vi "NEO Set Pod Setpoints.vi"(6 "Operation":T2, 8 "Steer Angles (degrees)":T3, 9 "Drive Velocities (ft/s)":T3, 10 "Pod Setpoints (ft/s and deg)":T16, 11 "Swerve Drive":T5={"Drive Motors (NEO)"={"Left Front"={"DeviceStatus"={"status"=FALSE, "code"=0, "source"=""}, "Type"=enum."PWM", "PWM"={"PWM Channel"=enum."Invalid", "DeadBand"={"Name"="", "maxPositivePwm"=0, "minPositivePwm"=0, "centerPwm"=0, "maxNegativePwm"=0, "minNegativePwm"=0, "angularRange"=0}}, "CAN"={"Device Number"=0, "SetOutput VI Ref"=variant, "GetOutput VI Ref"=variant, "Enable VI Ref"=variant, "Disable VI Ref"=variant, "Data"=variant}, "Invert"=FALSE, "DIO PWM"={"PWM \"Enable\" Channel"=enum."Invalid", "DIOChannel"=enum."Invalid", "PWM Rate"=0.0}}, "Left Back"={"DeviceStatus"={"status"=FALSE, "code"=0, "source"=""}, "Type"=enum."PWM", "PWM"={"PWM Channel"=enum."Invalid", "DeadBand"={"Name"="", "maxPositivePwm"=0, "minPositivePwm"=0, "centerPwm"=0, "maxNegativePwm"=0, "minNegativePwm"=0, "angularRange"=0}}, "CAN"={"Device Number"=0, "SetOutput VI Ref"=variant, "GetOutput VI Ref"=variant, "Enable VI Ref"=variant, "Disable VI Ref"=variant, "Data"=variant}, "Invert"=FALSE, "DIO PWM"={"PWM \"Enable\" Channel"=enum."Invalid", "DIOChannel"=enum."Invalid", "PWM Rate"=0.0}}, "Right Front"={"DeviceStatus"={"status"=FALSE, "code"=0, "source"=""}, "Type"=enum."PWM", "PWM"={"PWM Channel"=enum."Invalid", "DeadBand"={"Name"="", "maxPositivePwm"=0, "minPositivePwm"=0, "centerPwm"=0, "maxNegativePwm"=0, "minNegativePwm"=0, "angularRange"=0}}, "CAN"={"Device Number"=0, "SetOutput VI Ref"=variant, "GetOutput VI Ref"=variant, "Enable VI Ref"=variant, "Disable VI Ref"=variant, "Data"=variant}, "Invert"=FALSE, "DIO PWM"={"PWM \"Enable\" Channel"=enum."Invalid", "DIOChannel"=enum."Invalid", "PWM Rate"=0.0}}, "Right Back"={"DeviceStatus"={"status"=FALSE, "code"=0, "source"=""}, "Type"=enum."PWM", "PWM"={"PWM Channel"=enum."Invalid", "DeadBand"={"Name"="", "maxPositivePwm"=0, "minPositivePwm"=0, "centerPwm"=0, "maxNegativePwm"=0, "minNegativePwm"=0, "angularRange"=0}}, "CAN"={"Device Number"=0, "SetOutput VI Ref"=variant, "GetOutput VI Ref"=variant, "Enable VI Ref"=variant, "Disable VI Ref"=variant, "Data"=variant}, "Invert"=FALSE, "DIO PWM"={"PWM \"Enable\" Channel"=enum."Invalid", "DIOChannel"=enum."Invalid", "PWM Rate"=0.0}}}, "Steer Motors (NEO)"={"Left Front"={"DeviceStatus"={"status"=FALSE, "code"=0, "source"=""}, "Type"=enum."PWM", "PWM"={"PWM Channel"=enum."Invalid", "DeadBand"={"Name"="", "maxPositivePwm"=0, "minPositivePwm"=0, "centerPwm"=0, "maxNegativePwm"=0, "minNegativePwm"=0, "angularRange"=0}}, "CAN"={"Device Number"=0, "SetOutput VI Ref"=variant, "GetOutput VI Ref"=variant, "Enable VI Ref"=variant, "Disable VI Ref"=variant, "Data"=variant}, "Invert"=FALSE, "DIO PWM"={"PWM \"Enable\" Channel"=enum."Invalid", "DIOChannel"=enum."Invalid", "PWM Rate"=0.0}}, "Left Back"={"DeviceStatus"={"status"=FALSE, "code"=0, "source"=""}, "Type"=enum."PWM", "PWM"={"PWM Channel"=enum."Invalid", "DeadBand"={"Name"="", "maxPositivePwm"=0, "minPositivePwm"=0, "centerPwm"=0, "maxNegativePwm"=0, "minNegativePwm"=0, "angularRange"=0}}, "CAN"={"Device Number"=0, "SetOutput VI Ref"=variant, "GetOutput VI Ref"=variant, "Enable VI Ref"=variant, "Disable VI Ref"=variant, "Data"=variant}, "Invert"=FALSE, "DIO PWM"={"PWM \"Enable\" Channel"=enum."Invalid", "DIOChannel"=enum."Invalid", "PWM Rate"=0.0}}, "Right Front"={"DeviceStatus"={"status"=FALSE, "code"=0, "source"=""}, "Type"=enum."PWM", "PWM"={"PWM Channel"=enum."Invalid", "DeadBand"={"Name"="", "maxPositivePwm"=0, "minPositivePwm"=0, "centerPwm"=0, "maxNegativePwm"=0, "minNegativePwm"=0, "angularRange"=0}}, "CAN"={"Device Number"=0, "SetOutput VI Ref"=variant, "GetOutput VI Ref"=variant, "Enable VI Ref"=variant, "Disable VI Ref"=variant, "Data"=variant}, "Invert"=FALSE, "DIO PWM"={"PWM \"Enable\" Channel"=enum."Invalid", "DIOChannel"=enum."Invalid", "PWM Rate"=0.0}}, "Right Back"={"DeviceStatus"={"status"=FALSE, "code"=0, "source"=""}, "Type"=enum."PWM", "PWM"={"PWM Channel"=enum."Invalid", "DeadBand"={"Name"="", "maxPositivePwm"=0, "minPositivePwm"=0, "centerPwm"=0, "maxNegativePwm"=0, "minNegativePwm"=0, "angularRange"=0}}, "CAN"={"Device Number"=0, "SetOutput VI Ref"=variant, "GetOutput VI Ref"=variant, "Enable VI Ref"=variant, "Disable VI Ref"=variant, "Data"=variant}, "Invert"=FALSE, "DIO PWM"={"PWM \"Enable\" Channel"=enum."Invalid", "DIOChannel"=enum."Invalid", "PWM Rate"=0.0}}}, "Pigeon2"={"DeviceStatus"={"status"=FALSE, "code"=0, "source"=""}, "Device Number"=0, "Type"=352321536, "Device ID"=0, "Handle"=0, "UsageFrame"=0, "Library Path"=path ""}, "Radii (ft)"={"Left Front Position"=[], "Left Back Position"=[], "Right Front Position"=[], "Right Back Position"=[]}} {"Radii (ft)"."Right Back Position" format="%.2f"; "Radii (ft)"."Right Front Position" format="%.2f"; "Radii (ft)"."Left Back Position" format="%.2f"; "Radii (ft)"."Left Front Position" format="%.2f"; "Pigeon2"."Type" items=["CAN"=352321536, "TalonSRX"=33554432]}) -> ()   [LabVIEW 2023]
uses:
  Type Definitions/Data/Pod Setpoints.ctl
  Type Definitions/Hardware/Swerve Drives/(NEO-NEO-ThroughBore-Pigeon2) Swerve.ctl
  Type Definitions/Hardware/4 Motor Sets/(NEO & NEO 550) 4 Motor Set.ctl
  <vilib>/Rock Robotics/WPI/MotorControl/WPI_MotorControlDeviceRef.ctl
  <vilib>/Rock Robotics/WPI/MotorControl/WPI_MotorControlType.ctl
  <vilib>/Rock Robotics/SystemInterfaces/DIO/FPGA_DIOPWMChannel.ctl
  <vilib>/Rock Robotics/WPI/PWM/WPI_PWMDeadband.ctl
  <vilib>/Rock Robotics/SystemInterfaces/DIO/FPGA_DIOChannel.ctl
  <vilib>/Rock Robotics/WPI/ThirdParty/Phoenix-LabVIEW/Pigeon IMU/CTRE_PigeonIMU_DeviceRef.ctl
  <vilib>/Rock Robotics/WPI/ThirdParty/Phoenix-LabVIEW/Pigeon IMU/CTRE_PigeonIMU_ConnectionType.ctl
  Type Definitions/Data/Pod Positions.ctl
  Robot Code/Drive/Implementation/Drive Operations.ctl
  <vilib>/Rock Robotics/WPI/ThirdParty/REV Robotics/REVLib/Typedef/Spark MAX Control Type.ctl
  4b768f86-8279-4062-bf26-12cbbaf62c6c.vi
panel:
  out "Arbitrary":T1
  in  "PID Constants":T4={"P Gain"=0.0, "I Gain"=0.0, "D Gain"=0.0, "F Gain"=0.0, "I Zone"=0.0, "Min Output"=-1.0, "Max Output"=1.0}
  in  "Motor Type":enum16{"Drive", "Steer"}(ring)
  in  "Motor Position":T15(ring)
  out "PID Graph":cluster{"Left Front":dbl, "Theta":dbl}(graph)
  out "Values":cluster{"Actual":dbl, "Setpoint":dbl}
  in  "Debug Mode?":bool
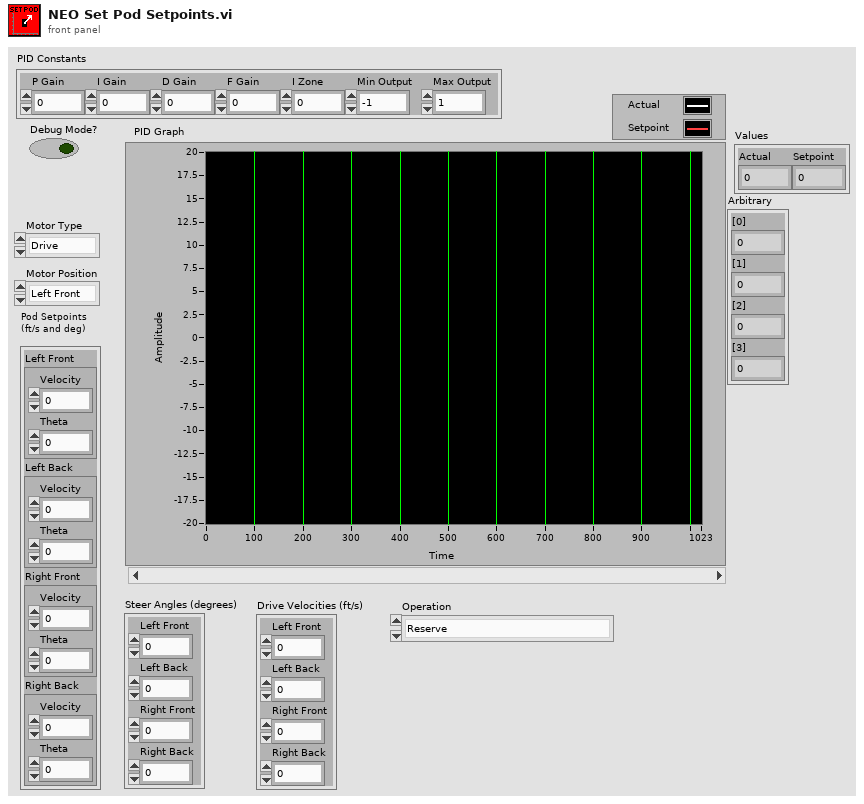
[diagram p1: front panel]
types:
  T1 = cluster{"[0]":dbl, "[1]":dbl, "[2]":dbl, "[3]":dbl}
  T2 = typedef "Drive Operations.ctl" = enum16{"Reserve", "Read Current", "Immediate", "Calibrate", "Auto"}
  T3 = cluster{"Left Front":dbl, "Left Back":dbl, "Right Front":dbl, "Right Back":dbl}
  T4 = cluster{"P Gain":dbl, "I Gain":dbl, "D Gain":dbl, "F Gain":dbl, "I Zone":dbl, "Min Output":dbl, "Max Output":dbl}
  T5 = typedef "(NEO-NEO-ThroughBore-Pigeon2) Swerve.ctl" = cluster{"Drive Motors (NEO)":T6, "Steer Motors (NEO)":T6, "Pigeon2":T12, "Radii (ft)":T14}
  T6 = typedef "(NEO & NEO 550) 4 Motor Set.ctl" = cluster{"Left Front":T7, "Left Back":T7, "Right Front":T7, "Right Back":T7}
  T7 = typedef "WPI_MotorControlDeviceRef.ctl" = cluster{"DeviceStatus":errorcluster, "Type":T8, "PWM":cluster{"PWM Channel":T9, "DeadBand":T10}, "CAN":cluster{"Device Number":u8, "SetOutput VI Ref":variant, "GetOutput VI Ref":variant, "Enable VI Ref":variant, "Disable VI Ref":variant, "Data":variant}, "Invert":bool, "DIO PWM":cluster{"PWM \"Enable\" Channel":T9, "DIOChannel":T11, "PWM Rate":dbl}}
  T8 = typedef "WPI_MotorControlType.ctl" = enum16{"PWM", "CAN", "DIO PWM"}
  T9 = typedef "FPGA_DIOPWMChannel.ctl" = enum8{"PWM 0", "PWM 1", "PWM 2", "PWM 3", "PWM 4", "PWM 5", "PWM 6", "PWM 7", "PWM 8", "PWM 9", "PWM MXP 0", "PWM MXP 1", "PWM MXP 2", "PWM MXP 3", "PWM MXP 4", "PWM MXP 5", "PWM MXP 6", "PWM MXP 7", "PWM MXP 8", "PWM MXP 9", "Invalid"}
  T10 = typedef "WPI_PWMDeadband.ctl" = cluster{"Name":string, "maxPositivePwm":i32, "minPositivePwm":i32, "centerPwm":i32, "maxNegativePwm":i32, "minNegativePwm":i32, "angularRange":u16}
  T11 = typedef "FPGA_DIOChannel.ctl" = enum8{"DIO 0", "DIO 1", "DIO 2", "DIO 3", "DIO 4", "DIO 5", "DIO 6", "DIO 7", "DIO 8", "DIO 9", "DIO MXP 0", "DIO MXP 1", "DIO MXP 2", "DIO MXP 3", "DIO MXP 4", "DIO MXP 5", "DIO MXP 6", "DIO MXP 7", "DIO MXP 8", "DIO MXP 9", "DIO MXP 10", "DIO MXP 11", "DIO MXP 12", "DIO MXP 13", "DIO MXP 14", "DIO MXP 15", "SPI Port CS1", "SPI Port CS2", "SPI Port CS3", "SPI Port MISO", "SPI Port MOSI", "Invalid"}
  T12 = typedef "CTRE_PigeonIMU_DeviceRef.ctl" = cluster{"DeviceStatus":errorcluster, "Device Number":u8, "Type":T13, "Device ID":u32, "Handle":u64, "UsageFrame":u32, "Library Path":path}
  T13 = typedef "CTRE_PigeonIMU_ConnectionType.ctl" = u32
  T14 = typedef "Pod Positions.ctl" = cluster{"Left Front Position":dbl[], "Left Back Position":dbl[], "Right Front Position":dbl[], "Right Back Position":dbl[]}
  T15 = enum16{"Left Front", "Left Back", "Right Front", "Right Back"}
  T16 = typedef "Pod Setpoints.ctl" = cluster{"Left Front":cluster{"Velocity":dbl, "Theta":dbl}, "Left Back":cluster{"Velocity":dbl, "Theta":dbl}, "Right Front":cluster{"Velocity":dbl, "Theta":dbl}, "Right Back":cluster{"Velocity":dbl, "Theta":dbl}}
  T17 = typedef "Spark MAX Control Type.ctl" = enum16{"Percent VBus", "Voltage", "Velocity", "Position", "Smart Motion", "Current", "Smart Velocity", "MAXMotion Position", "MAXMotion Velocity"}
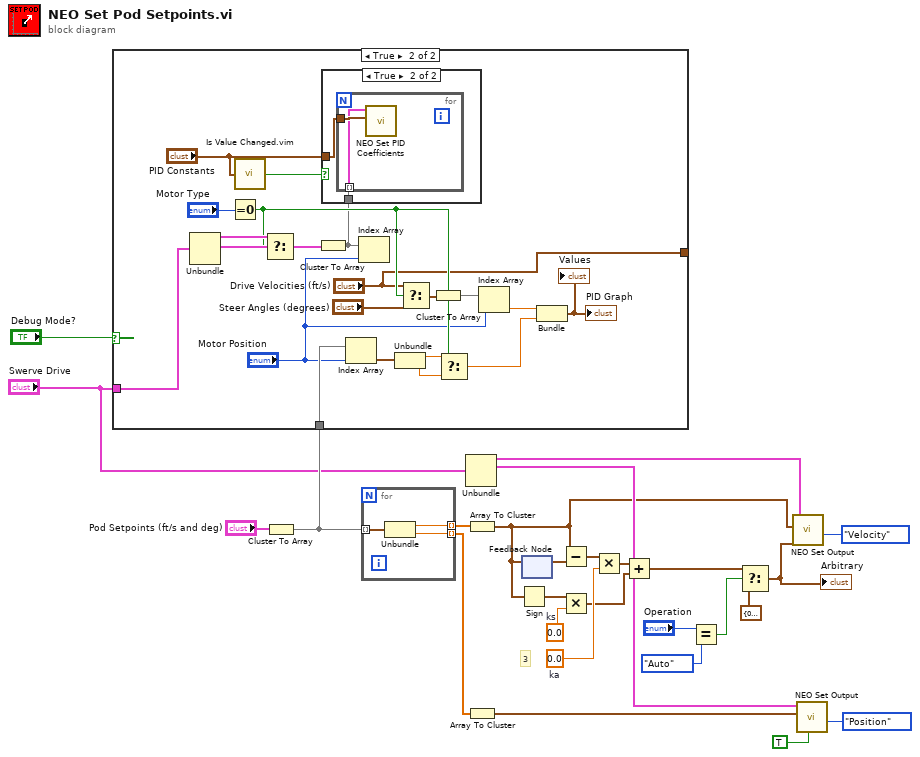
[diagram p0: block diagram]
diagram:
  w16 = 0.0  # ks
  w19 = 0.0  # ka
  # "3"
  n1 = Cluster To Array(cluster="Pod Setpoints (ft/s and deg)") -> (array=w24:cluster{"Velocity":dbl, "Theta":dbl}[])
  n2 = case shown="True" "Debug Mode?" {
    tunnel: "Swerve Drive" -> [_ w33]
    tunnel: w24 -> [_ w35]
    tunnel: [_ "Drive Velocities (ft/s)"] -> _
    frame False {
    }
    frame True {
      n3 = Unbundle(w33) -> ("Drive Motors (NEO)"=w46:T6, "Steer Motors (NEO)"=w45:T6)  [unwired: 2 out]
      n4 = Equal To 0?(x="Motor Type") -> (x = 0?=w40:bool)
      n5 = call "Is Value Changed.vim"("value"="PID Constants") -> ("changed or first call?"=w28:bool)
      n6 = Select(t=w46, s=w40, f=w45) -> (s? t:f=w32:T6)
      n7 = Cluster To Array(cluster=w32) -> (array=w27:T7[])
      n8 = case shown="True" w28 {
        tunnel: "PID Constants" -> [_ w49]
        tunnel: w27 -> [_ w48]
        frame False {
        }
        frame True {
          n9 = for {
            tunnel: w49 -> [w51]
            tunnel: w48 -> [w50] mode=indexing
            n10 = call "NEO Set PID Coefficients.vi"("PID Constants"=w51, "MotorControlDeviceRef in"=w50) -> ()  [unwired: 6 in, 2 out]
          }
        }
      }
      n11 = Index Array(array=w35, index="Motor Position") -> (element=w44:cluster{"Velocity":dbl, "Theta":dbl})
      n12 = Index Array(array=w27, index="Motor Position") -> ()  [unwired: 1 out]
      n13 = Unbundle(w44) -> ("Velocity"=w43:dbl, "Theta"=w42:dbl)
      n14 = Select(t="Drive Velocities (ft/s)", s=w40, f="Steer Angles (degrees)") -> (s? t:f=w39:T3)
      n15 = Cluster To Array(cluster=w39) -> (array=w38:dbl[])
      n16 = Select(t=w43, s=w40, f=w42) -> (s? t:f=w36:dbl)
      n17 = Index Array(array=w38, index="Motor Position") -> (element=w37:dbl)
      n18 = Bundle("Left Front"=w37, "Theta"=w36) -> (→"PID Graph" →"Values":cluster{"Left Front":dbl, "Theta":dbl})  [unwired: 1 in]
    }
  }
  n19 = for {
    tunnel: w24 -> [w54] mode=indexing
    tunnel: [w53] -> w23 mode=indexing
    tunnel: [w52] -> w22 mode=indexing
    n20 = Unbundle(w54) -> ("Velocity"=w53:dbl, "Theta"=w52:dbl)
  }
  n21 = Unbundle("Swerve Drive") -> ("Drive Motors (NEO)"=w21:T6, "Steer Motors (NEO)"=w14:T6)  [unwired: 2 out]
  n22 = Array To Cluster(array=w23) -> (cluster=w4:T1)
  n23 = Array To Cluster(array=w22) -> (cluster=w5:T1)
  n24 = Sign(1:w4) -> (0:w17:T1)
  n25 = feedback #1() -> (w20:T1)  [unwired: 1 in]
  n26 = feedback-in #1(w4) -> ()
  n27 = Subtract(x=w4, y=w20) -> (x-y=w13:T1)
  n28 = Multiply(x=w17, y=w16) -> (x*y=w15:T1)
  n29 = Multiply(x=w13, y=w19) -> (x*y=w18:T1)
  n30 = Add(x=w18, y=w15) -> (x+y=w11:T1)
  n31 = Equal?(x="Operation", y=Drive_Operations."Auto") -> (x = y?=w6:bool)
  n32 = Select(t=w11, s=w6, f=T1 {"[0]"=0.0, "[1]"=0.0, "[2]"=0.0, "[3]"=0.0}) -> (s? t:f=w8:T1)
  "Arbitrary" <- w8
  n33 = call "NEO Set Output.vi"("Arbitrary Feedforward"=w8, "Control Mode"=Spark_MAX_Control_Type."Velocity", "Setpoints"=w4, "Motors"=w21) -> ()  [unwired: 8 in]
  n34 = call "NEO Set Output.vi"("Add Angle Offsets?"=TRUE, "Control Mode"=Spark_MAX_Control_Type."Position", "Setpoints"=w5, "Motors"=w14) -> ()  [unwired: 8 in]
